vi "Controller_Adrian.vi"(0 "name 2":string, 5 "port or service name":u16=16389, 7 "connection ID":refnum<k16>, 9 "error in (no error)":errorcluster, 11 "x":sgl[](array[numeric])) -> (4 "*(type *) &x":dbl[](array[numeric]), 6 "error out":errorcluster, 8 "connection ID out":refnum<k16>)   [LabVIEW 2021]
panel:
  out "error in (no error) 2":errorcluster
  out "error out 2":errorcluster
  out "error IO":errorcluster
  out "port":u16
  out "name":string
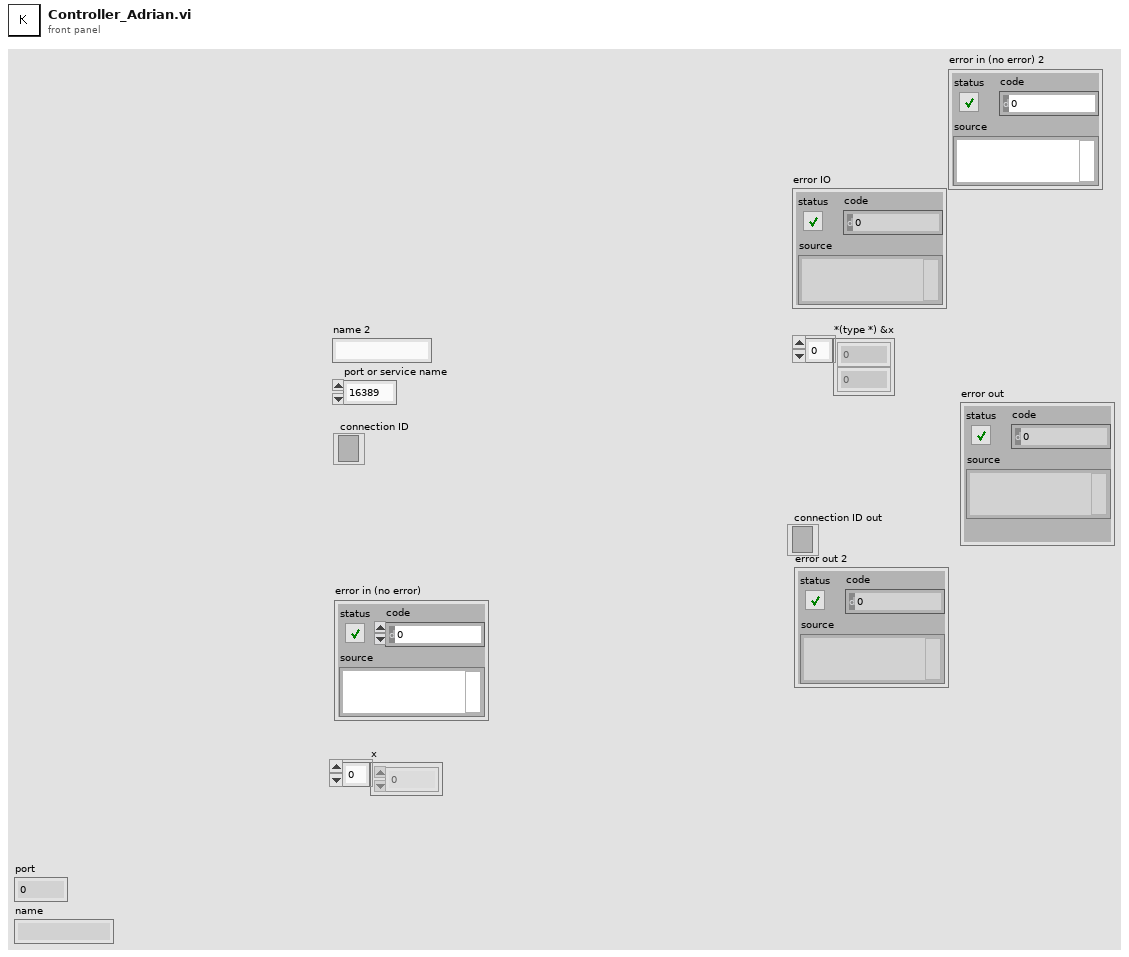
[diagram p1: front panel]
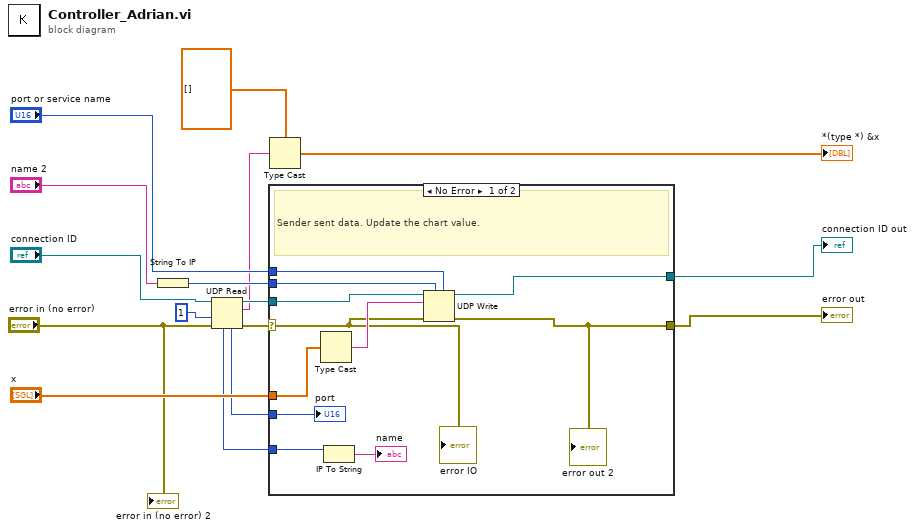
[diagram p0: block diagram]
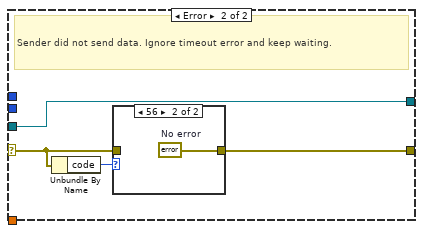
[diagram p2: hidden frame]
diagram:
  n1 = String To IP(1:"name 2") -> (0:w3:u32)
  n2 = UDP Read(connection ID="connection ID", timeout ms (25000)=1, 8:"error in (no error)") -> (data out=w1:string, error out=w7:errorcluster, 3:w4:refnum<k16>, 4:w6:u16, 6:w5:u32)  [unwired: 1 out]
  n3 = case shown="No Error" w7 {
    selector: w7 -> [w18 w30]
    tunnel: [w17 w28] -> w11
    tunnel: [w27 w29] -> w10
    tunnel: w6 -> [w25 _]
    tunnel: w5 -> [w24 _]
    tunnel: w4 -> [w23 w29]
    tunnel: "port or service name" -> [w22 _]
    tunnel: w3 -> [w21 _]
    tunnel: "x" -> [w19 _]
    frame No Error {
      # "Sender sent data. Update the chart value."
      n4 = Type Cast(x=w19) -> (*(type *) &x=w20:string)  [unwired: 1 in]
      n5 = IP To String(2:w24) -> (0:→"name":string)  [unwired: 1 in]
      n6 = UDP Write(address=w21, port or service name=w22, connection ID=w23, data in=w20, 8:w18) -> (error out=w17:errorcluster, 3:w27:refnum<k16>)  [unwired: 1 in]
      "error out 2" <- w17
      "port" <- w25
      "error IO" <- w18
    }
    frame Error {
      # "Sender did not send data. Ignore timeout error and keep waiting."
      n7 = Unbundle By Name(w30) -> ("code"=w31:i32)
      n8 = case shown="56" w31 {
        tunnel: w30 -> [w32 _]
        tunnel: [w32 w33] -> w28
        frame Default {
        }
        frame 56 {
          w33 = errorcluster {"status"=FALSE, "code"=0, "source"=""}  # No error
        }
      }
    }
  }
  "error out" <- w11
  "connection ID out" <- w10
  n9 = Type Cast(type=dbl[] [], x=w1) -> (*(type *) &x=→"*(type *) &x":dbl[])
  "error in (no error) 2" <- "error in (no error)"
